vi "TAT_Read MAC.vi"(8 "error in (no error)":errorcluster) -> (0 "error out":errorcluster, 2 "MAC2":string, 3 "MAC1":string)   [LabVIEW 2017]
panel:
  out "standard output":string
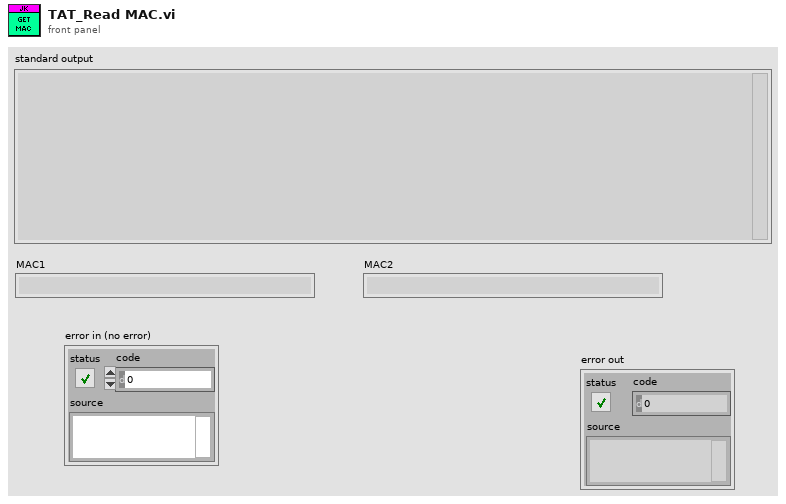
[diagram p1: front panel]
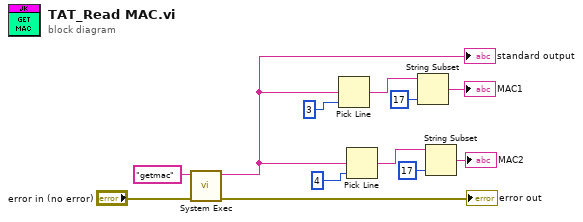
[diagram p0: block diagram]
diagram:
  n1 = call <vilib>:"System Exec.vi"("error in (no error)"="error in (no error)", "command line"="getmac") -> ("error out"=→"error out":errorcluster, "standard output"=w2:string)  [unwired: 6 in, 2 out]
  "standard output" <- w2
  n2 = Pick Line(multi-line string=w2, line index=3) -> (output string=w8:string)  [unwired: 1 in]
  n3 = Pick Line(multi-line string=w2, line index=4) -> (output string=w3:string)  [unwired: 1 in]
  n4 = String Subset(string=w8, length (rest)=17 ("length (rest)")) -> (substring=→"MAC1":string)  [unwired: 1 in]
  n5 = String Subset(string=w3, length (rest)=17 ("length (rest)")) -> (substring=→"MAC2":string)  [unwired: 1 in]
